vi "MyDaq_Task.vi"(8 "error in (no error)":errorcluster, 11 "Device + Encoder Channel":tag="myDAQ1/ctr0") -> (0 "error out":errorcluster, 3 "Refnum out":refnum<k21>)   [LabVIEW 2018]
doc: "This VI creates a channel which comes from myDAQ and then configures parameters of the signal such as the rising/falling pulse, etc and starts the task.\n\n\nInputs:\nError in.\n\nOutputs:\nRefunm out;\nError out."
uses:
  <vilib>/DAQmx/create/channels.llb/DAQmx Create Channel (CI-Count Edges).vi
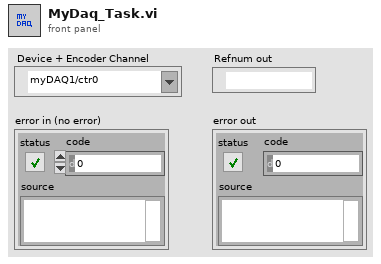
[diagram p1: front panel]
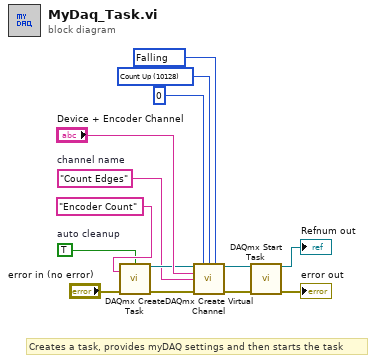
[diagram p0: block diagram]
diagram:
  w9 = 10128 items=["Count Up"=10128, "Count Down"=10124, "Externally Controlled"=10326] ("count direction")
  w8 = 10171 items=["Rising"=10280, "Falling"=10171] ("Edge")
  w1 = "Count Edges"  # channel name
  w3 = TRUE  # auto cleanup
  # "Creates a task, provides myDAQ settings and then starts the task"
  n1 = call <vilib>:"DAQmx Create Task.vi"("new task name"="Encoder Count", "auto cleanup"=w3, "error in"="error in (no error)") -> ("task out"=w2:refnum<k21>, "error out"=w4:errorcluster)  [unwired: 11 in]
  n2 = call-poly <vilib>:"DAQmx Create Virtual Channel.vi"("task in"=w2, "initial count"=u32 0, "count direction"=w9, "edge"=w8, "counter"="Device + Encoder Channel", "name to assign"=w1, "error in"=w4) -> ("task out"=w6:refnum<k21>, "error out"=w5:errorcluster)  [unwired: 7 in]
  n3 = call <vilib>:"DAQmx Start Task.vi"("task/channels in"=w6, "error in"=w5) -> ("task out"=→"Refnum out":refnum<k21>, "error out"=→"error out":errorcluster)  [unwired: 12 in]
